vi "getXmlNode.vi"(8 "error in (no error)":errorcluster, 11 "SettingsManager.lvclass in":refnum<class "SettingsManager.lvclass">) -> (0 "error out":errorcluster, 2 "xmlNode":refnum<class "xmlNode.lvclass">, 3 "SettingsManager.lvclass out":refnum<class "SettingsManager.lvclass">)   [LabVIEW 2011, in "Tools.lvlib" / "Settings.lvlib" / "SettingsManager.lvclass"]
uses:
  SettingsManager.lvclass
  xmlNode/xmlNode.lvclass
  SettingsManager.lvclass/SettingsManager.ctl
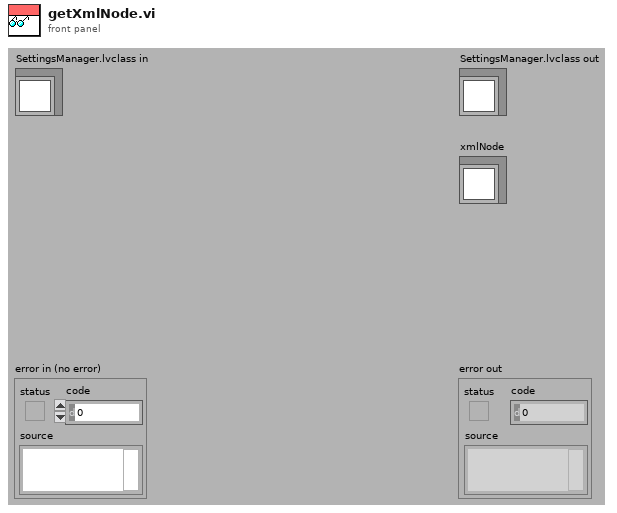
[diagram p1: front panel]
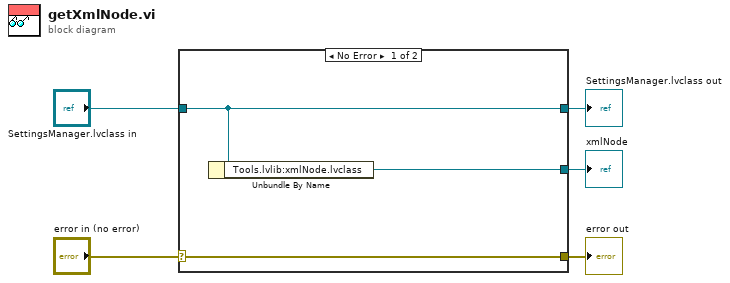
[diagram p0: block diagram]
diagram:
  n1 = case shown="No Error" "error in (no error)" {
    selector: "error in (no error)" -> [w8 w9]
    tunnel: [w8 w9] -> w4
    tunnel: [w7 w10] -> w2
    tunnel: "SettingsManager.lvclass in" -> [w7 w10]
    tunnel: [w6 _] -> w1
    frame No Error {
      n2 = Unbundle By Name(w7) -> ("Tools.lvlib:xmlNode.lvclass"=w6:refnum<class "xmlNode.lvclass">)
    }
    frame Error {
    }
  }
  "error out" <- w4
  "SettingsManager.lvclass out" <- w2
  "xmlNode" <- w1
